vi "Set startup speed.vi"(8 "error in (no error)":errorcluster, 11 "StageSPIM in":refnum<class "StageSPIM.lvclass">) -> (0 "error out":errorcluster, 3 "StageSPIM out":refnum<class "StageSPIM.lvclass">)   [LabVIEW 2012, in "StageSPIM.lvclass"]
uses:
  StageSPIM.lvclass
  StageSPIM.lvclass/StageSPIM.ctl
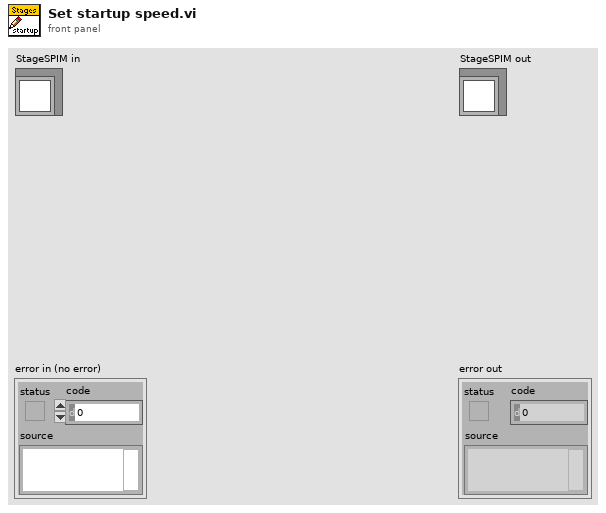
[diagram p1: front panel]
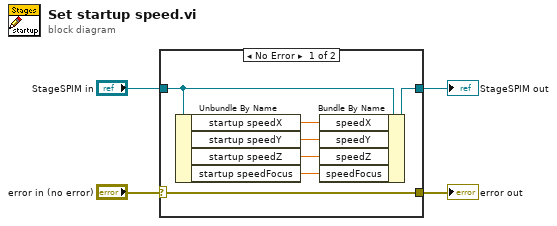
[diagram p0: block diagram]
diagram:
  n1 = case shown="No Error" "error in (no error)" {
    selector: "error in (no error)" -> [w11 w13]
    tunnel: [w11 w13] -> w3
    tunnel: [w9 w12] -> w1
    tunnel: "StageSPIM in" -> [w10 w12]
    frame No Error {
      n2 = Unbundle By Name(w10) -> ("startup speedX"=w8:dbl[unit], "startup speedY"=w7:dbl[unit], "startup speedZ"=w6:dbl[unit], "startup speedFocus"=w5:dbl[unit])
      n3 = Bundle By Name(cluster=w10, "speedX"=w8, "speedY"=w7, "speedZ"=w6, "speedFocus"=w5) -> (w9:refnum<class "StageSPIM.lvclass">)
    }
    frame Error {
    }
  }
  "error out" <- w3
  "StageSPIM out" <- w1
